vi "Global Stop.vi"() -> ()   [LabVIEW 2012]
panel:
  in  "Stop?":bool
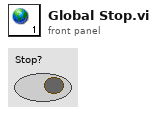
[diagram p1: front panel]
diagram:
